vi "Add Hardware.vi"(8 "error in (no error)":errorcluster, 10 "new plugin":refnum<class "Generic Plugin.lvclass">, 11 "Plugin Array in":refnum<class "Controller Array.lvclass">) -> (0 "error out":errorcluster, 3 "Plugin Array out":refnum<class "Controller Array.lvclass">)   [LabVIEW 2020, in "RxnRover.lvlib"]
doc: "Adds the reactor component plugin to the plugin list."
uses:
  RxnRover.lvlib
  Controller Array/Controller Array.lvclass
  Controller/Generic Plugin.lvclass
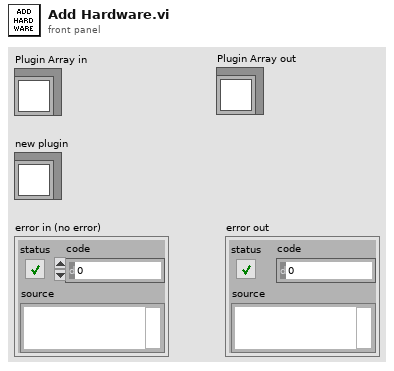
[diagram p1: front panel]
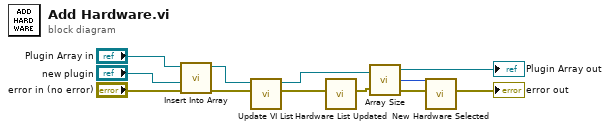
[diagram p0: block diagram]
diagram:
  n1 = call "Insert Into Array.vi"("error in (no error)"="error in (no error)", "new element"="new plugin", "Controller Array in"="Plugin Array in") -> ("error out"=w11:errorcluster, "Controller Array out"=w10:refnum<class "Controller Array.lvclass">)  [unwired: 2 in, 1 out]
  n2 = call "Update VI List.vi"("error in (no error)"=w11, "Controller Array in"=w10) -> ("error out"=w12:errorcluster, "Controller Array out"=w5:refnum<class "Controller Array.lvclass">)  [unwired: 8 in]
  n3 = call "Hardware List Updated.vi"("error in (no error)"=w12) -> ("error out"=w8:errorcluster)  [unwired: 10 in]
  n4 = call "Array Size.vi"("Controller Array in"=w5, "error in (no error)"=w8) -> ("Controller Array out"=→"Plugin Array out":refnum<class "Controller Array.lvclass">, "size(s)"=w6:i32, "error out"=w7:errorcluster)
  n5 = call "New Hardware Selected.vi"("error in (no error)"=w7, "Hardware Index"=w6) -> ("error out"=→"error out":errorcluster)  [unwired: 9 in]
